vi "Layer ID Extractor.vi"(8 "Error In":errorcluster, 11 "Layer Data":variant[][](array[variant])=[[variant]]) -> (0 "Error Out":errorcluster, 3 "Layer ID":i32)   [LabVIEW 2020]
uses:
  <vilib>/addons/database/_DB Variant To Data/Database Variant To Data.xnode
panel:
  out "data":string[][](array[string])
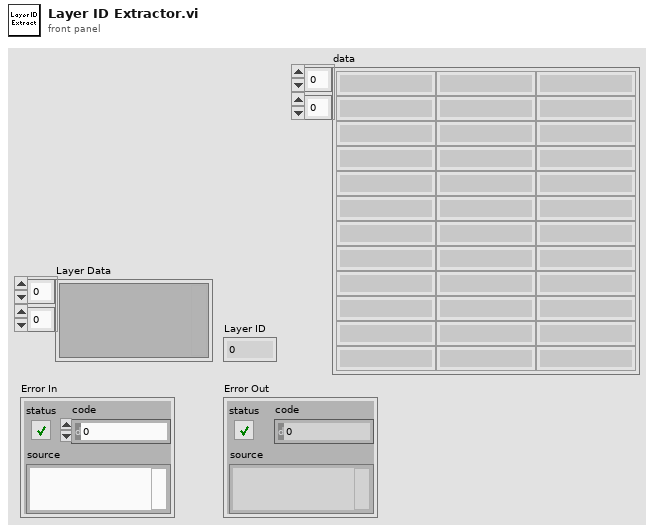
[diagram p1: front panel]
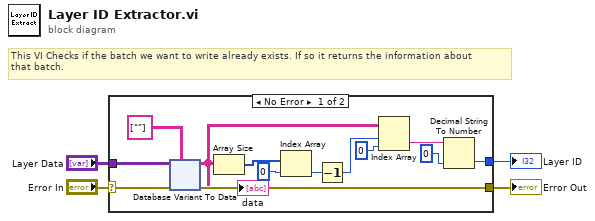
[diagram p0: block diagram]
diagram:
  # "This VI Checks if the batch we want to write already exists. If so it returns the information about\nthat batch."
  n1 = case shown="No Error" "Error In" {
    selector: "Error In" -> [w15 w62]
    tunnel: "Layer Data" -> [w16 _]
    tunnel: [w14 w62] -> w2
    tunnel: [w5 _] -> w1
    frame No Error {
      n2 = xnode "Database Variant To Data"("database variant"=w16, "error in (no error)"=w15, "type"=string[][] [[""]] ("columns")) -> ("data"=w9:string[][], "error out"=w14:errorcluster)
      "data" <- w9
      n3 = Array Size(array=w9) -> (size(s)=w13:i32[])
      n4 = Index Array(array=w13, index=0) -> (element=w11:i32)
      n5 = Decrement(x=w11) -> (x-1=w10:i32)
      n6 = Index Array(array=w9, index (row)=w10, index (col)=0 ("disabled index (col)")) -> (element=w7:string)
      n7 = Decimal String To Number(string=w7, default (0L)=0 ("default (0 I32)")) -> (number=w5:i32)  [unwired: 1 in, 1 out]
    }
    frame Error {
    }
  }
  "Error Out" <- w2
  "Layer ID" <- w1
